vi "Actor Core.vi"(8 "error in":errorcluster, 11 "Iterator Actor in":refnum<class "Abstract Iterator Actor.lvclass">) -> (0 "error out":errorcluster, 3 "Actor out":refnum<class "Actor.lvclass">)   [LabVIEW 2021, in "Iterator Actor.lvlib" / "Abstract Iterator Actor.lvclass"]
doc: "(<B>Filename</B>: Actor Framework.lvlib:Actor.lvclass:Actor Core.vi)\n\nReceives messages to the actor, reacts to them, and initiates any error handling that may shut the actor down.\n\nDescendant classes may override this VI to append parallel tasks for the actor to complete while it handles messages. Overrides use the Call Parent Method node."
uses:
  Abstract Iterator Actor.lvclass
  C:/Program Files/National Instruments/LabVIEW 2021/vi.lib/ActorFramework/Actor/Actor.lvclass
  <vilib>/ActorFramework/Actor/Actor.lvclass
  Abstract Iterator Actor.lvclass/Abstract Iterator Actor.ctl
  Iterator Settings.ctl
  Active Stop Conditions.ctl
  <vilib>/ActorFramework/Message/Message.lvclass
  Iterator Actor/Iterator Actor Abstract Messages/Iterator Report Iterations End Msg/Iterator Report Iterations End Msg.lvclass
  <vilib>/ActorFramework/Actor/Actor.lvclass/Actor.ctl
  <vilib>/ActorFramework/Message Enqueuer/Message Enqueuer.lvclass/Message Enqueuer.ctl
  Stop Reason.ctl
  <vilib>/ActorFramework/Message Enqueuer/Init from Existing Queue.vi
  <vilib>/MGI/Monitored Actor/Monitored Actor/Monitored Actor/Monitored Actor.lvclass
  <vilib>/ActorFramework/Message Enqueuer/Message Enqueuer.lvclass
  Iterator Actor/Iterator Actor Messages/Report Iterations End Msg/Report Iterations End Msg.lvclass
  Iterator Actor/Iterator Actor Messages/Write Stop Reason Msg/Write Stop Reason Msg.lvclass
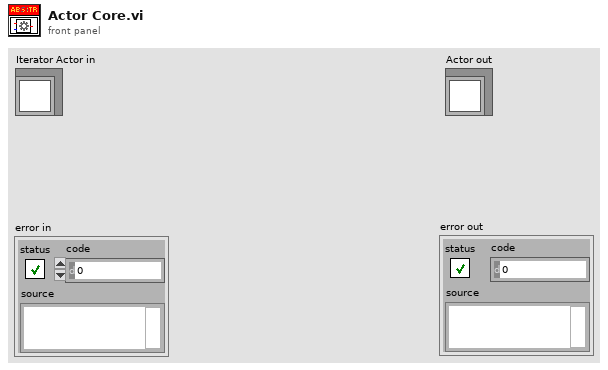
[diagram p1: front panel]
types:
  T1 = typedef "Iterator Actor.lvlib/Abstract Iterator Actor.lvclass/Iterator Settings.ctl" = cluster{"Prepare timeout (ms)":i32, "Iterate timeout (ms)":i32, "Conclude timeout (ms)":i32, "Iterate period (ms)":i32, "Number of iterations":i32, "Time before stop (ms)":i32, "Active Stop Conditions":T2, "Prepare Msg":refnum<class "Message.lvclass">, "Iterate Msg":refnum<class "Message.lvclass">, "Conclude Msg":refnum<class "Message.lvclass">, "Iterations End Report":refnum<class "Iterator Report Iterations End Msg.lvclass">}
  T2 = typedef "Iterator Actor.lvlib/Abstract Iterator Actor.lvclass/Active Stop Conditions.ctl" = cluster{"Number of Iterations":bool, "Time Elapsed":bool, "Iteration Result":bool}
  T3 = typedef "Iterator Actor.lvlib/Abstract Iterator Actor.lvclass/Stop Reason.ctl" = enum16{"Number of Iterations", "Time Elapsed", "Stopped Internally", "Stopped Externally"}
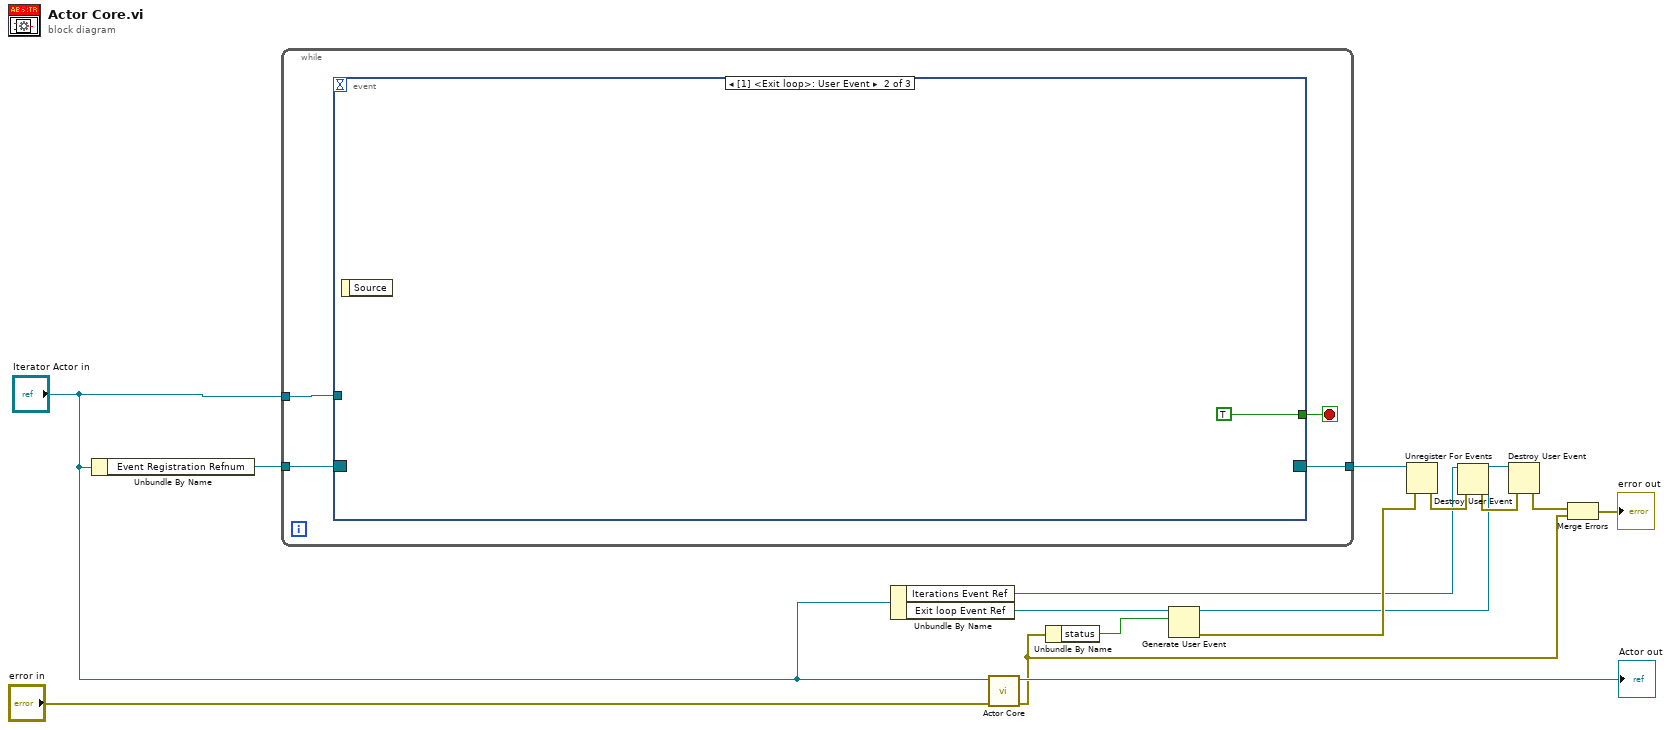
[diagram p0: block diagram]
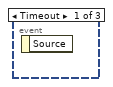
[diagram p2: hidden frame]
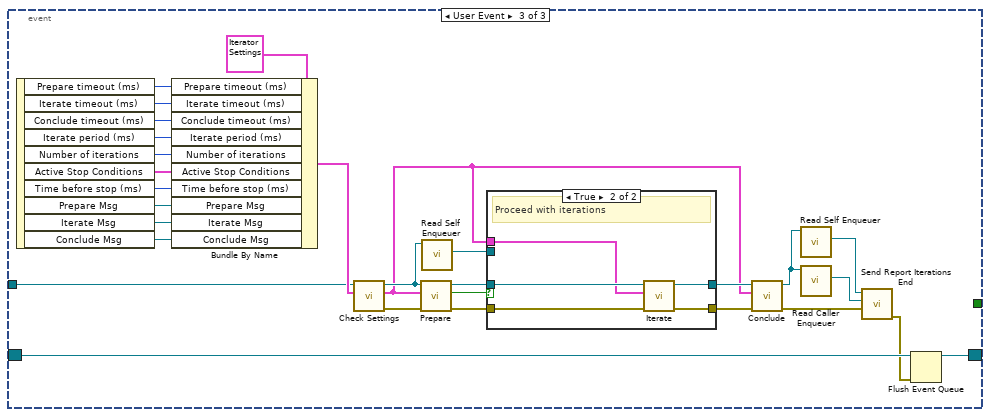
[diagram p3: hidden frame]
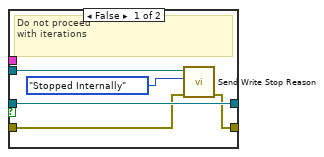
[diagram p4: hidden frame]
diagram:
  n1 = Unbundle By Name("Iterator Actor in") -> ("Event Registration Refnum"=w2:refnum<event-registration>)
  n2 = while {
    tunnel: w2 -> [w19]
    tunnel: [w17] -> w12
    tunnel: "Iterator Actor in" -> [w16]
    stop <- w18 stop-if-true
    n3 = event shown="[1] <Exit loop>: User Event" {
      selector: w19 -> [_ _ w31]
      dyn-events: [_ _ w32] -> w17
      timeout: _ -> [_ _ _]
      tunnel: [_ TRUE _] -> w18
      tunnel: w16 -> [_ _ w26]
      event Timeout {
        n4 = event-data() -> ()  [unwired: 1 in, 1 out]
      }
      event User Event {
        n5 = event-data() -> ()  [unwired: 1 in, 1 out]
      }
      event User Event {
        n6 = event-data() -> ("Prepare timeout (ms)"=w47:i32, "Iterate timeout (ms)"=w46:i32, "Conclude timeout (ms)"=w45:i32, "Iterate period (ms)"=w44:i32, "Number of iterations"=w43:i32, "Active Stop Conditions"=w28:T2, "Time before stop (ms)"=w42:i32, "Prepare Msg"=w41:refnum<class "Message.lvclass">, "Iterate Msg"=w40:refnum<class "Message.lvclass">, "Conclude Msg"=w39:refnum<class "Message.lvclass">)  [unwired: 1 in]
        n7 = Bundle By Name(cluster=T1 {"Prepare timeout (ms)"=0, "Iterate timeout (ms)"=0, "Conclude timeout (ms)"=0, "Iterate period (ms)"=0, "Number of iterations"=0, "Time before stop (ms)"=0, "Active Stop Conditions"={"Number of Iterations"=FALSE, "Time Elapsed"=FALSE, "Iteration Result"=FALSE}, "Prepare Msg"=refnum, "Iterate Msg"=refnum, "Conclude Msg"=refnum, "Iterations End Report"=refnum} ("Iterator Settings"), "Prepare timeout (ms)"=w47, "Iterate timeout (ms)"=w46, "Conclude timeout (ms)"=w45, "Iterate period (ms)"=w44, "Number of iterations"=w43, "Active Stop Conditions"=w28, "Time before stop (ms)"=w42, "Prepare Msg"=w41, "Iterate Msg"=w40, "Conclude Msg"=w39) -> (w33:T1)
        n8 = call-dynamic "Check Settings.vi"("Iterator Settings in"=w33, "Abstract Iterator Actor in"=w26) -> ("error out"=w34:errorcluster, "Iterator Settings out"=w21:T1, "Abstract Iterator Actor out"=w22:refnum<class "Abstract Iterator Actor.lvclass">)  [unwired: 7 in]
        n9 = call-dynamic "Prepare.vi"("error in"=w34, "Iterator Settings"=w21, "Abstract Iterator Actor in"=w22) -> ("error out"=w35:errorcluster, "Reply"=w36:bool, "Abstract Iterator Actor out"=w38:refnum<class "Abstract Iterator Actor.lvclass">)  [unwired: 6 in]
        n10 = call <vilib>:"Read Self Enqueuer.vi"("Actor"=w22) -> ("Self Enqueuer"=w24:refnum<class "Message Enqueuer.lvclass">)  [unwired: 10 in]
        n11 = case shown="True" w36 {
          tunnel: [w52 w59] -> w49
          tunnel: w21 -> [_ w55]
          tunnel: w38 -> [w54 w58]
          tunnel: [w54 w57] -> w37
          tunnel: w35 -> [w53 w56]
          tunnel: w24 -> [w51 _]
          frame False {
            # "Do not proceed \nwith iterations"
            n12 = call "Send Write Stop Reason.vi"("error in (no error)"=w53, "Stop Reason"=Stop_Reason."Stopped Internally", "Message Enqueuer in"=w51) -> ("error out"=w52:errorcluster)  [unwired: 7 in, 1 out]
          }
          frame True {
            # "Proceed with iterations"
            n13 = call-dynamic "Iterate.vi"("error in (no error)"=w56, "Iterator Settings"=w55, "Abstract Iterator Actor in"=w58) -> ("error out"=w59:errorcluster, "Abstract Iterator Actor out"=w57:refnum<class "Abstract Iterator Actor.lvclass">)  [unwired: 7 in]
          }
        }
        n14 = call-dynamic "Conclude.vi"("error in (no error)"=w49, "Iterator Settings"=w21, "Abstract Iterator Actor in"=w37) -> ("error out"=w29:errorcluster, "Abstract Iterator Actor out"=w25:refnum<class "Abstract Iterator Actor.lvclass">)  [unwired: 7 in]
        n15 = call <vilib>:"Read Self Enqueuer.vi"("Actor"=w25) -> ("Self Enqueuer"=w23:refnum<class "Message Enqueuer.lvclass">)  [unwired: 10 in]
        n16 = call <vilib>:"Read Caller Enqueuer.vi"("Actor"=w25) -> ("Caller Enqueuer"=w27:refnum<class "Message Enqueuer.lvclass">)  [unwired: 10 in]
        n17 = call "Send Report Iterations End.vi"("Iterator Error"=w29, "Caller Enqueuer in"=w27, "Message Enqueuer in"=w23) -> ("error out"=w30:errorcluster)  [unwired: 7 in, 1 out]
        n18 = Flush Event Queue(0:w31, 3:w30) -> (8:w32:refnum<event-registration>)  [unwired: 4 in, 2 out]
      }
    }
  }
  n19 = Unbundle By Name("Iterator Actor in") -> ("Iterations Event Ref"=w6:refnum<user-event>, "Exit loop Event Ref"=w14:refnum<user-event>)
  n20 = call-parent "Actor Core.vi"("error in"="error in", "Actor in"="Iterator Actor in") -> ("error out"=w4:errorcluster, "Actor out"=→"Actor out":refnum<class "Actor.lvclass">)  [unwired: 8 in]
  n21 = Unbundle By Name(w4) -> ("status"=w3:bool)
  n22 = Generate User Event(user event=w14, event data cluster=w3) -> (user event out=w7:refnum<user-event>, error out=w10:errorcluster)  [unwired: 2 in]
  n23 = Unregister For Events(event registration refnum=w12, error in=w10) -> (error out=w11:errorcluster)
  n24 = Destroy User Event(user event=w6, error in=w11) -> (error out=w9:errorcluster)
  n25 = Destroy User Event(user event=w7, error in=w9) -> (error out=w8:errorcluster)
  n26 = Merge Errors(w8, w4) -> (→"error out":errorcluster)
